vi "Rename Item By Name.vi"(8 "error in (no error)":errorcluster, 9 "New Name":string, 10 "Old Name":string, 11 "Parent Ref in":T1 format="%.0x") -> (0 "error out":errorcluster, 2 "Item Ref out":T1 format="%.0x", 3 "Parent Ref out":T1 format="%.0x")   [LabVIEW 2015, in "Chassis TimeSync System Explorer.lvlib"]
uses:
  Chassis TimeSync System Explorer.lvlib
  <vilib>/NI Veristand/Custom Device API/Custom Device Item Ref.ctl
  <vilib>/NI Veristand/Custom Device API/Custom Device API.lvlib
  <vilib>/NI Veristand/Custom Device Tools/Custom Device Utility Library/Custom Device Utility Library.lvlib
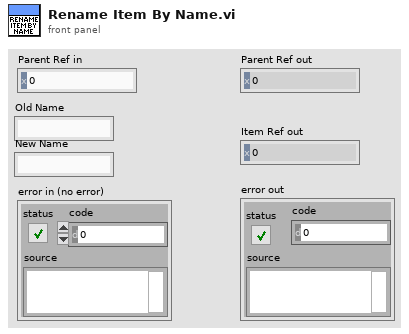
[diagram p1: front panel]
types:
  T1 = typedef "Custom Device API.lvlib/Custom Device Item Ref.ctl" = u64
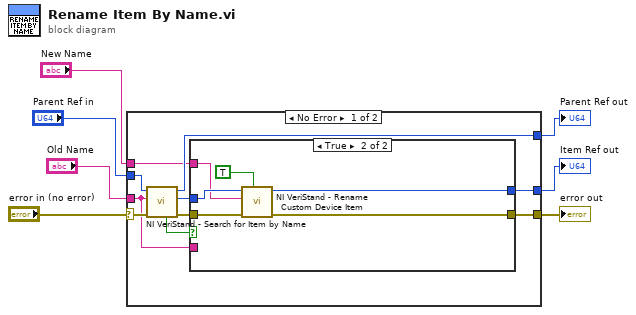
[diagram p0: block diagram]
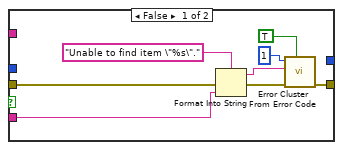
[diagram p2: hidden frame]
diagram:
  n1 = case shown="No Error" "error in (no error)" {
    selector: "error in (no error)" -> [w13 w33]
    tunnel: "Parent Ref in" -> [w15 w32]
    tunnel: [w12 w33] -> w5
    tunnel: [w11 w32] -> w4
    tunnel: "Old Name" -> [w10 _]
    tunnel: "New Name" -> [w9 _]
    tunnel: [w8 _] -> w1
    frame No Error {
      n2 = call <vilib>:"NI VeriStand - Search for Item by Name.vi"("error in"=w13, "Item Name"=w10, "Section Ref in"=w15) -> ("error out"=w14:errorcluster, "Item Ref"=w16:T1, "Section Ref out"=w11:T1, "Found"=w17:bool)  [unwired: 5 in]
      n3 = case shown="True" w17 {
        tunnel: w16 -> [_ w30]
        tunnel: w14 -> [w23 w29]
        tunnel: [w25 w26] -> w12
        tunnel: w10 -> [w20 _]
        tunnel: w9 -> [_ w28]
        tunnel: [_ w27] -> w8
        frame False {
          n4 = Format Into String(format string="Unable to find item \"%s\"." ("error message (\"\")"), error in=w23, w20) -> (resulting string=w22:string, error out=w21:errorcluster)  [unwired: 1 in]
          n5 = call <vilib>:"Error Cluster From Error Code.vi"("show call chain? (False)"=TRUE, "error in (no error)"=w21, "error message (\"\")"=w22, "error code (0)"=1) -> ("error out"=w25:errorcluster)  [unwired: 5 in]
        }
        frame True {
          n6 = call <vilib>:"NI VeriStand - Rename Custom Device Item.vi"("Force Rename (F)"=TRUE, "error in (no error)"=w29, "New Name"=w28, "Item Ref in"=w30) -> ("error out"=w26:errorcluster, "Item Ref out"=w27:T1)  [unwired: 5 in, 1 out]
        }
      }
    }
    frame Error {
    }
  }
  "error out" <- w5
  "Item Ref out" <- w1
  "Parent Ref out" <- w4
